vi "Power Meter Front Panel.vi"() -> ()   [LabVIEW 2009]
doc: "Front Panel for Newport 1830-C power meter."
uses:
  Newport 1830-C/Newport 1830-C.lvlib
panel:
  in  "Read to Controls":bool
  out "Units (1:4)":i32
  out "AVG (1:3)":i32
  out "Run/Stop (1:0)":i32
  out "ATTN (0:1)":i32
  out "Local Lockout (0:1)":i32
  out "Zero (0:1)":i32
  out "Beeper (0:1)":i32
  out "Backlight (0:2)":i32
  out "Range (1:8)":i32
  out "Wavelength (nnnn)":i32
  in  "Read Count":i32=1
  out "SI Power":string
  out "Power":dbl
  out "error code out":i32 format="%0.0f"
  in  "Read":bool caption="Read to Controls"
  in  "Read Power":bool
  in  "Set":bool
  in  "Run/Stop":u16(ring) items=["Stop", "Run"]
  in  "Wavelength":i32
  in  "stop":bool
  in  "ATTN":u16(ring) items=["Off", "On"]
  in  "BKLT":u16(ring) items=["Off", "Low", "High"]
  in  "Range":i32(ring) items=["Auto", "Lowest", "2", "3", "4", "5", "6", "7", "Highest"]
  in  "Beep":u16(ring) items=["Off", "On"]
  in  "AVG":i32(ring) items=["Slow"=1, "Medium"=2, "Fast"=3]
  in  "Store\nReference":bool
  in  "Units":i32(ring) items=["W"=1, "dB"=2, "mdB"=3, "REL"=4]
  in  "Zero":u16(ring) items=["Off", "On"]
  in  "Local":u16(ring) items=["Off", "On"]
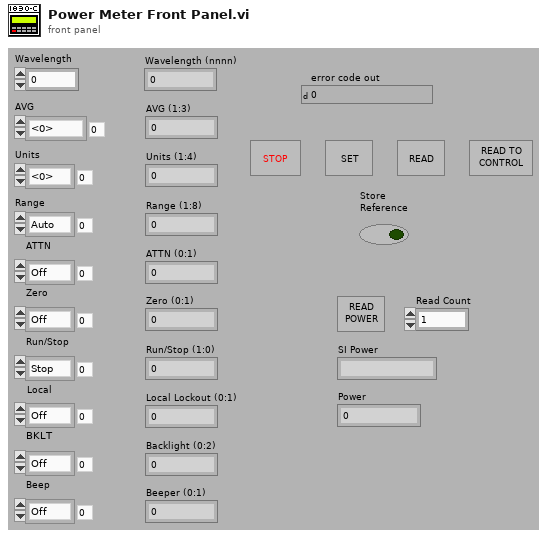
[diagram p1: front panel]
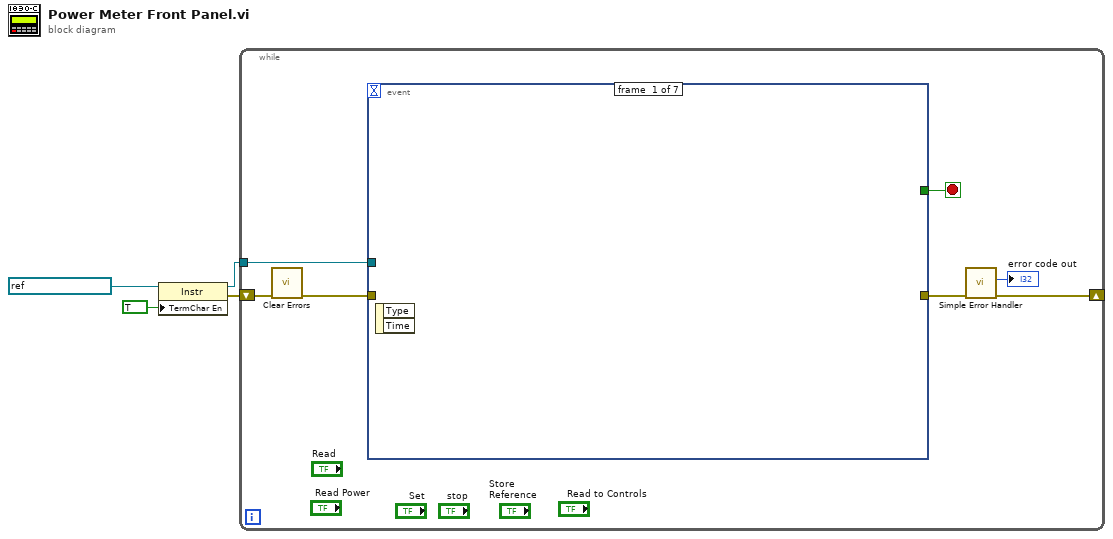
[diagram p0: block diagram]
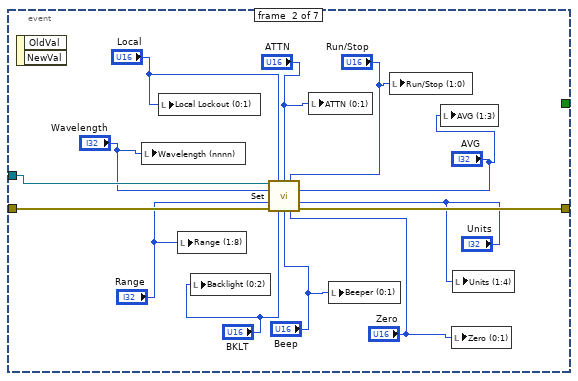
[diagram p2: hidden frame]
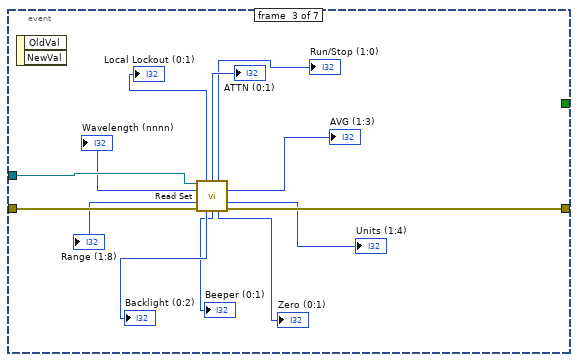
[diagram p3: hidden frame]
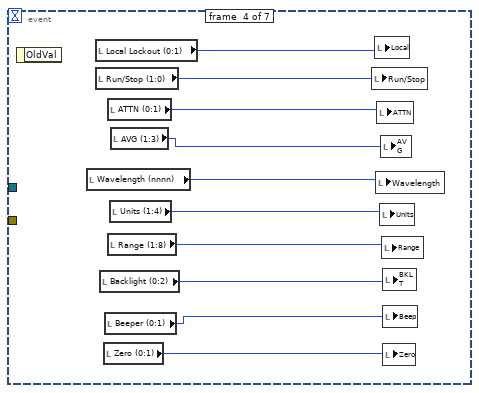
[diagram p4: hidden frame]
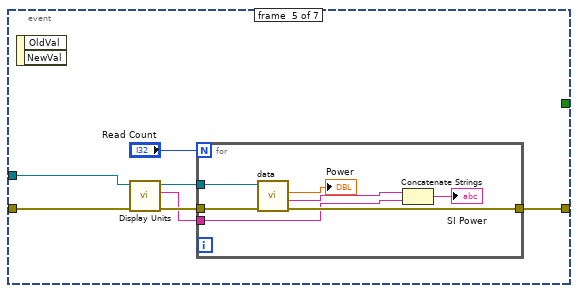
[diagram p5: hidden frame]
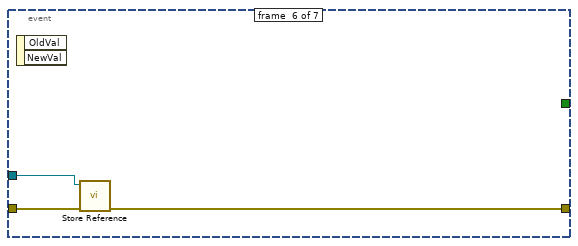
[diagram p6: hidden frame]
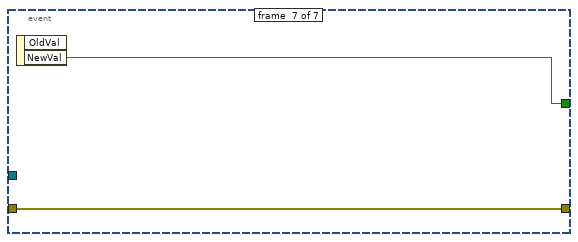
[diagram p7: hidden frame]
diagram:
  n1 = property class="Instr"(reference=refnum<visa-resource-name> "GPIB::4::INSTR" ("VISA resource name"), "TermChar En"=TRUE ("Message Based Settings:Termination Character Enable")) -> (reference out=w3:refnum<visa-resource-name>, error out=w2:errorcluster)  [unwired: 1 in]
  n2 = while {
    shift-right: [w11] -> _
    shift-left: w2 -> [w10]
    tunnel: w3 -> [w6]
    stop <- w8 stop-if-true
    n3 = call <vilib>:"Clear Errors.vi"("error in (no error)"=w10) -> ("error out"=w5:errorcluster)  [unwired: 6 in]
    n4 = event shown="[5] \"Store\nReference\": Value Change" {
      selector: _ -> [_ _ _ _ _ _ _]
      dyn-events: _ -> [_ _ _ _ _ _ _]
      timeout: _ -> [_ _ _ _ _ _ _]
      tunnel: w6 -> [_ w23 w37 _ w53 w64 _]
      tunnel: w5 -> [_ w24 w36 _ w52 w63 w65]
      tunnel: [_ w22 w35 _ w54 w62 w65] -> w9
      tunnel: [_ _ _ _ _ _ w66] -> w8
      event #0 {
        n5 = event-data() -> ()  [unwired: 1 in, 2 out]
      }
      event #1 {
        n6 = event-data() -> ()  [unwired: 1 in, 2 out]
        n7 = local write "Wavelength (nnnn)"("Wavelength") -> ()
        n8 = local write "Local Lockout (0:1)"("Local") -> ()
        n9 = local write "Range (1:8)"("Range") -> ()
        n10 = local write "Backlight (0:2)"("BKLT") -> ()
        n11 = call "Set.vi"("VISA resource name"=w23, "Local Lockout (0:1)"="Local", "ATTN (0:1)"="ATTN", "Run/Stop (1:0)"="Run/Stop", "Wavelength (nnnn)"="Wavelength", "AVG (1:3)"="AVG", "Range (0-Auto,1:8)"="Range", "Units (1:4)"="Units", "error in (no error)"=w24, "Backlight (0:2)"="BKLT", "Beeper (0:1)"="Beep", "Zero (0:1)"="Zero") -> ("error out"=w22:errorcluster)  [unwired: 2 in, 1 out]
        n12 = local write "ATTN (0:1)"("ATTN") -> ()
        n13 = local write "Beeper (0:1)"("Beep") -> ()
        n14 = local write "Run/Stop (1:0)"("Run/Stop") -> ()
        n15 = local write "AVG (1:3)"("AVG") -> ()
        n16 = local write "Zero (0:1)"("Zero") -> ()
        n17 = local write "Units (1:4)"("Units") -> ()
      }
      event #2 {
        n18 = event-data() -> ()  [unwired: 1 in, 2 out]
        n19 = call "Read Set.vi"("VISA resource name"=w37, "error in (no error)"=w36) -> ("Local Lockout (0:1)"=→"Local Lockout (0:1)":i32, "ATTN (0:1)"=→"ATTN (0:1)":i32, "Run/Stop (1:0)"=→"Run/Stop (1:0)":i32, "Wavelength (nnnn)"=→"Wavelength (nnnn)":i32, "AVG (1:3)"=→"AVG (1:3)":i32, "Range (1:8)"=→"Range (1:8)":i32, "Units (1:4)"=→"Units (1:4)":i32, "Backlight (0:2)"=→"Backlight (0:2)":i32, "Beeper (0:1)"=→"Beeper (0:1)":i32, "Zero (0:1)"=→"Zero (0:1)":i32, "error out"=w35:errorcluster)  [unwired: 2 in, 1 out]
      }
      event #3 {
        n20 = event-data() -> ()  [unwired: 1 in, 1 out]
        n21 = local read "Wavelength (nnnn)"() -> (w43:i32)
        n22 = local read "Local Lockout (0:1)"() -> (w47:i32)
        n23 = local read "Run/Stop (1:0)"() -> (w46:i32)
        n24 = local read "Backlight (0:2)"() -> (w40:i32)
        n25 = local read "Zero (0:1)"() -> (w38:i32)
        n26 = local read "Beeper (0:1)"() -> (w39:i32)
        n27 = local read "ATTN (0:1)"() -> (w45:i32)
        n28 = local read "Range (1:8)"() -> (w41:i32)
        n29 = local read "Units (1:4)"() -> (w42:i32)
        n30 = local read "AVG (1:3)"() -> (w44:i32)
        n31 = local write "Run/Stop"(w46) -> ()
        n32 = local write "Local"(w47) -> ()
        n33 = local write "Wavelength"(w43) -> ()
        n34 = local write "ATTN"(w45) -> ()
        n35 = local write "Units"(w42) -> ()
        n36 = local write "AVG"(w44) -> ()
        n37 = local write "Range"(w41) -> ()
        n38 = local write "BKLT"(w40) -> ()
        n39 = local write "Beep"(w39) -> ()
        n40 = local write "Zero"(w38) -> ()
      }
      event #4 {
        n41 = event-data() -> ()  [unwired: 1 in, 2 out]
        n42 = call "Display Units.vi"("error in (no error)"=w52, "VISA resource name"=w53) -> ("error out"=w50:errorcluster, "Units"=w49:string, "VISA resource name out"=w51:refnum<visa-resource-name>)  [unwired: 7 in]
        n43 = for {
          N: "Read Count" -> [_]
          tunnel: w51 -> [w61]
          tunnel: w50 -> [w60]
          tunnel: [w59] -> w54
          tunnel: w49 -> [w57]
          n44 = call "data.vi"("error in (no error)"=w60, "VISA resource name"=w61) -> ("error out"=w59:errorcluster, "SI"=w56:string, "output"=→"Power":dbl)  [unwired: 6 in, 1 out]
          n45 = Concatenate Strings(w56, w57) -> (→"SI Power":string)
        }
      }
      event #5 {
        n46 = event-data() -> ()  [unwired: 1 in, 2 out]
        n47 = call "Store Reference.vi"("error in (no error)"=w63, "VISA resource name"=w64) -> ("error out"=w62:errorcluster)  [unwired: 8 in, 1 out]
      }
      event #6 {
        n48 = event-data() -> ("NewVal"=w66:bool)  [unwired: 1 in, 1 out]
      }
    }
    n49 = call <vilib>:"Simple Error Handler.vi"("error in (no error)"=w9) -> ("code out"=→"error code out":i32, "error out"=w11:errorcluster)  [unwired: 4 in, 3 out]
  }
